vi "nanomsg_bind.vi"(3 "error in":errorcluster, 4 "endpoint":string="tcp://", 5 "socket in":refnum<class "nanomsg_socket.lvclass">) -> (0 "error out":errorcluster, 2 "socket out":refnum<class "nanomsg_socket.lvclass">)   [LabVIEW 2014, in "nanomsg.lvlib" / "nanomsg_socket.lvclass"]
doc: "Bind a socket to a particular <b>endpoint</b>. This is somewhat similiar to \"listening\" for a connection.\n\nThe endpoint string specifies the protocol and the port to accept connection from. In this instance the originating host and port may each be wildcarded (*).\n\nExamples for \"endpoint\":\n tcp://localhost:1234\n tcp://*:5432\n inproc://namedprocess\n\nDetailed API documentation: http://nanomsg.org/documentation.html"
uses:
  nanomsg_socket.lvclass
  nanomsg_socket.lvclass/nanomsg_socket.ctl
  <vilib>/Utility/error.llb/Error Cluster From Error Code.vi
  nanomsg.lvlib
panel:
  # "NN"
  # "labview"
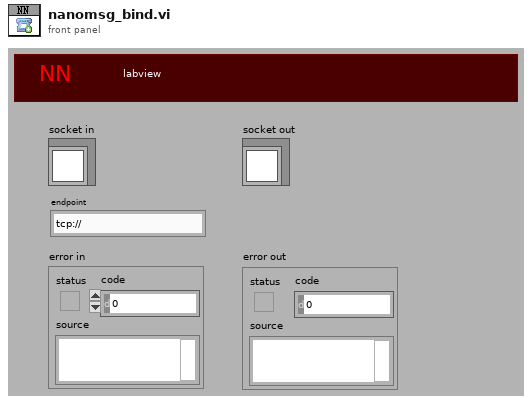
[diagram p1: front panel]
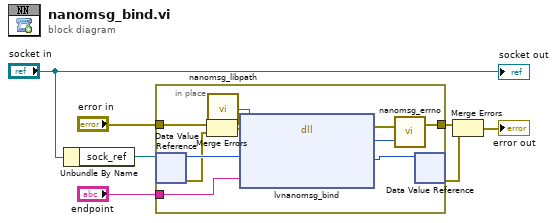
[diagram p0: block diagram]
diagram:
  n1 = Unbundle By Name("socket in") -> ("sock_ref"=w3:refnum<data-value>)
  n2 = in-place {
    in-place-border: "endpoint" -> [w17]
    in-place-border: "error in" -> [w16]
    in-place-border: [w13] -> w5
    n3 = in-place-dvr #1(w3) -> (w12:u64, w8:errorcluster)
    n4 = Merge Errors(w16, w8) -> (w9:errorcluster)
    n5 = call "nanomsg_libpath.vi"() -> ("path"=w10:path)
    n6 = dll-call lib="?" fn="lvnanomsg_bind" ("zmq_labview.dll:lvzmq_bind")(path in=w10, error in=w9, "sock_obj"=w12, "endpoint"=w17) -> (error out=w15:errorcluster, "return type"=w14:i32, "sock_obj"=w11:u64)  [unwired: 2 in, 1 out]
    n7 = call "nanomsg_errno.vi"("retval"=w14, "error in"=w15) -> ("error out"=w13:errorcluster)  [unwired: 1 out]
    n8 = in-place-dvr #1(w11) -> (w1:errorcluster)  [unwired: 1 out]
  }
  n9 = Merge Errors(w5, w1) -> (→"error out":errorcluster)
  "socket out" <- "socket in"
